vi "Connection Callback.vi"(7 "Owner":refnum<class>, 10 "Connection State":T1, 11 "Endpoint":refnum<class "Endpoint.lvclass">) -> ()   [LabVIEW 2020, in "LV Chat Server.lvclass"]
uses:
  LV Chat Server.lvclass
  <vilib>/IlluminatedG/lv-stream/Connection State.ctl
  <vilib>/IlluminatedG/lv-msg-simple/Stream-Simple-Msg/Endpoint/Endpoint.lvclass
  Data Types/Message ID.ctl
  LV Chat Server.lvclass/LV Chat Server.ctl
  User.ctl
  <vilib>/IlluminatedG/lv-stream/stream/Stream.lvclass/Stream.ctl
  e61c04f8-2e71-45c4-8a38-0e0d383b5b34.vi
  0747b19a-0b0c-467b-bdca-b12aa573beb4.vi
  <vilib>/IlluminatedG/lv-msg-simple/Stream-Simple-Msg/Endpoint/Write Flattened Data.vi
  0747b19a-0b0c-467b-bdca-b12aa573beb4.vi/2bb808b0-5d94-493e-a99c-e70b6b44e968.vi
  <vilib>/IlluminatedG/lv-stream/stream/Write Data.vi
  0747b19a-0b0c-467b-bdca-b12aa573beb4.vi/2bb808b0-5d94-493e-a99c-e70b6b44e968.vi/850aaa44-16cf-4b05-95d8-204edf60ad4b.vi
  <vilib>/IlluminatedG/lv-stream/stream/Dispatch Sniffer Data.vi
  <vilib>/IlluminatedG/lv-stream/stream/Prepared.vi
  <vilib>/IlluminatedG/lv-stream/Endpoint/Cast Sniffer Callback.vi
  <vilib>/IlluminatedG/lv-msg-simple/Stream-Simple-Msg/Endpoint/Get Format.vi
  <vilib>/IlluminatedG/lv-msg-simple/Stream-Simple-Msg/Endpoint/Get Stream.vi
  <vilib>/Utility/error.llb/Error Cluster From Error Code.vi
  <vilib>/IlluminatedG/lv-stream/stream/Stream.lvclass
  <vilib>/IlluminatedG/lv-stream/URI/URI.lvclass
  <vilib>/IlluminatedG/lv-stream/Stream.lvlib
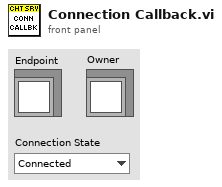
[diagram p1: front panel]
types:
  T1 = typedef "Stream.lvlib/Connection State.ctl" = enum16{"Connected", "Disconnected"}
  T2 = typedef "Message ID.ctl" = enum16{"UserInfo", "UserList", "Message", "Disconnect"}
  T3 = typedef "LV Chat Server.lvclass/User.ctl" = cluster{"Name":string, "IP":string, "Connected At":dbl, "Endpoint":refnum<class "Endpoint.lvclass">}
  T4 = typedef "LV Chat Server.lvclass/Ref Data.ctl" = cluster{"Endpoint Map":map{string, T3}, "User Map":map{string, string}}
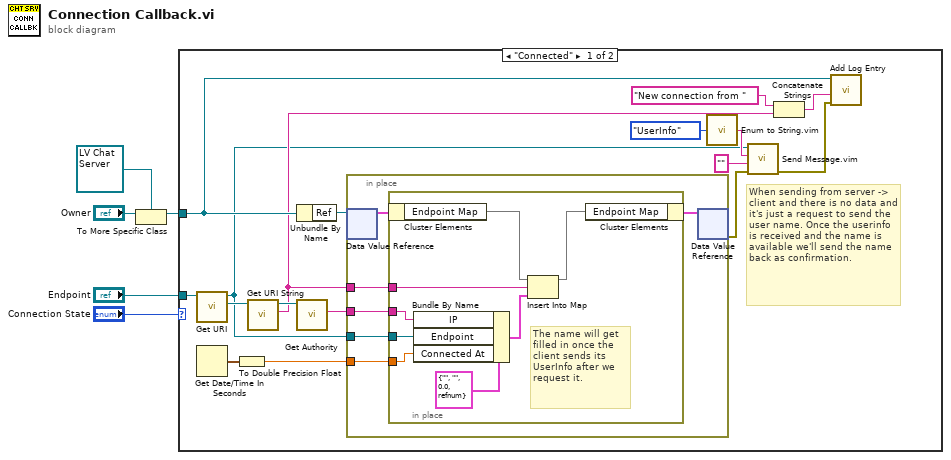
[diagram p0: block diagram]
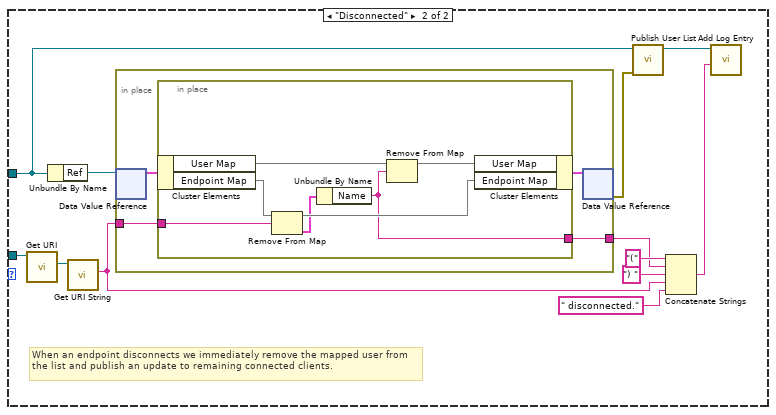
[diagram p2: hidden frame]
diagram:
  n1 = To More Specific Class(target class=refnum<class "LV Chat Server.lvclass"> refnum ("LV Chat Server.lvclass"), reference="Owner") -> (specific class reference=w1:refnum<class "LV Chat Server.lvclass">)  [unwired: 1 in, 1 out]
  n2 = case shown="\"Connected\"" "Connection State" {
    tunnel: "Endpoint" -> [w21 w47]
    tunnel: w1 -> [w10 w44]
    frame "Connected" {
      # "When sending from server -> client and there is no data and it's just a request to send the user name. Once the userinfo is received and the name is available we'll send the name back as confirmation."
      n3 = call <vilib>:"Get URI.vi"("Endpoint in"=w21) -> ("URI"=w20:refnum<class "URI.lvclass">, "Endpoint out"=w6:refnum<class "Endpoint.lvclass">)  [unwired: 8 in, 1 out]
      n4 = Get Date/Time In Seconds() -> (seconds since 1Jan1904=w17:timestamp)
      n5 = To Double Precision Float(number=w17) -> (double precision float=w16:dbl)
      n6 = call <vilib>:"Get URI String.vi"("URI in"=w20) -> ("URI String"=w9:string, "URI out"=w19:refnum<class "URI.lvclass">)  [unwired: 8 in, 1 out]
      n7 = Unbundle By Name(w10) -> ("Ref"=w22:refnum<data-value>)
      n8 = call <vilib>:"Get Authority.vi"("URI in"=w19) -> ("Authority"=w18:string)  [unwired: 8 in, 2 out]
      n9 = in-place {
        in-place-border: w9 -> [w26]
        in-place-border: w18 -> [w25]
        in-place-border: w16 -> [w24]
        in-place-border: w6 -> [w23]
        n10 = in-place-dvr #1(w22) -> (w28:T4)  [unwired: 1 out]
        n11 = in-place {
          in-place-border: w26 -> [w35]
          in-place-border: w25 -> [w32]
          in-place-border: w24 -> [w31]
          in-place-border: w23 -> [w30]
          # "The name will get filled in once the client sends its UserInfo after we request it."
          n12 = in-place-cluster #2(w28) -> ("Endpoint Map"=w36:map{string, T3})
          n13 = Bundle By Name(cluster=T3 {"Name"="", "IP"="", "Connected At"=0.0, "Endpoint"=refnum} ("value"), "IP"=w32, "Endpoint"=w30, "Connected At"=w31) -> (w33:T3)
          n14 = Insert Into Map(map in=w36, key=w35, value=w33) -> (map out=w29:map{string, T3})  [unwired: 2 out]
          n15 = in-place-cluster #2("Endpoint Map"=w29) -> (w27:T4)
        }
        n16 = in-place-dvr #1(w27) -> (w15:errorcluster)  [unwired: 1 out]
      }
      n17 = call "Enum to String.vim"("Enum"=Message_ID."UserInfo" ("Message ID")) -> ("Enum String"=w13:string)
      n18 = call "Send Message.vim"("error in (no error)"=w15, "Data"="", "ID"=w13, "Endpoint in"=w6) -> ("error out"=w8:errorcluster)  [unwired: 6 in, 1 out]
      n19 = Concatenate Strings("New connection from ", w9) -> (w11:string)
      n20 = call "Add Log Entry.vi"("error in (no error)"=w8, "Message"=w11, "LV Chat Server in"=w10) -> ()  [unwired: 7 in, 2 out]
    }
    frame "Disconnected" {
      # "When an endpoint disconnects we immediately remove the mapped user from the list and publish an update to remaining connected clients."
      n21 = call <vilib>:"Get URI.vi"("Endpoint in"=w47) -> ("URI"=w46:refnum<class "URI.lvclass">)  [unwired: 8 in, 2 out]
      n22 = Unbundle By Name(w44) -> ("Ref"=w48:refnum<data-value>)
      n23 = call <vilib>:"Get URI String.vi"("URI in"=w46) -> ("URI String"=w39:string)  [unwired: 8 in, 2 out]
      n24 = in-place {
        in-place-border: w39 -> [w50]
        in-place-border: [w49] -> w40
        n25 = in-place-dvr #3(w48) -> (w52:T4)  [unwired: 1 out]
        n26 = in-place {
          in-place-border: w50 -> [w58]
          in-place-border: [w53] -> w49
          n27 = in-place-cluster #4(w52) -> ("User Map"=w55:map{string, string}, "Endpoint Map"=w59:map{string, T3})
          n28 = Remove From Map(10:w58, 11:w59) -> (1:w56:T3, 3:w57:map{string, T3})  [unwired: 1 out]
          n29 = Unbundle By Name(w56) -> ("Name"=w53:string)
          n30 = Remove From Map(10:w53, 11:w55) -> (3:w54:map{string, string})  [unwired: 2 out]
          n31 = in-place-cluster #4("User Map"=w54, "Endpoint Map"=w57) -> (w51:T4)
        }
        n32 = in-place-dvr #3(w51) -> (w45:errorcluster)  [unwired: 1 out]
      }
      n33 = call "Publish User List.vi"("error in (no error)"=w45, "LV Chat Server in"=w44) -> ("LV Chat Server out"=w43:refnum<class "LV Chat Server.lvclass">)  [unwired: 8 in, 1 out]
      n34 = Concatenate Strings("(" ("string"), w40, ") " ("string"), w39, " disconnected." ("string")) -> (w37:string)
      n35 = call "Add Log Entry.vi"("Message"=w37, "LV Chat Server in"=w43) -> ()  [unwired: 8 in, 2 out]
    }
  }
